vi "Write Table Reference.vi"(10 "Table Reference":refnum<data-value>, 11 "LookupTable in":refnum<class "LookupTable.lvclass">) -> (3 "LookupTable out":refnum<class "LookupTable.lvclass">)   [LabVIEW 2017, in "LookupTable.lvlib" / "LookupTable.lvclass"]
uses:
  LookupTable.lvclass
  LookupTable.lvclass/LookupTable.ctl
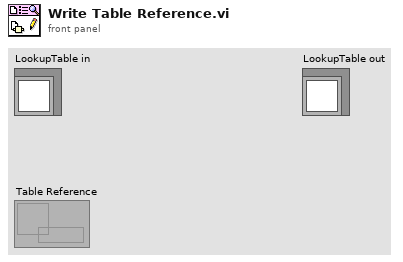
[diagram p1: front panel]
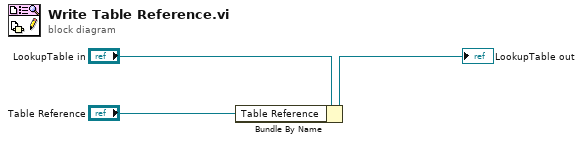
[diagram p0: block diagram]
diagram:
  n1 = Bundle By Name(cluster="LookupTable in", "Table Reference"="Table Reference") -> (→"LookupTable out":refnum<class "LookupTable.lvclass">)
